vi "Test Host.vi"() -> ()   [LabVIEW 2014]
uses:
  <vilib>/FPGAPlugInAG/PXIe-7962R/niLvFpga_Open_PXIe-7962R.vi
  <vilib>/rvi/interface/common/dynamic/niFpgaDynamicAddResources.vi
  <vilib>/LabVIEW Targets/FPGA/FlexRIO/CustomFPGAMethods/79XXR_Method_IOModuleStatusImpl.vi
  <vilib>/Utility/error.llb/Error Cluster From Error Code.vi
  <vilib>/rvi/errors/niLvFpgaAdjustHostInterfaceError.vi
  <vilib>/rvi/interface/common/niFpgaWaitOnOcc.vi
  <instrlib>/_niInstr/Streaming/v1/Host/Public/Start Finite Stream.vi
  <instrlib>/_niInstr/Streaming/v1/Host/Public/Wait for Stream.vi
  <vilib>/FPGAPlugInAG/Dynamic/niLvFpga_Close_Dynamic.vi
  <vilib>/rvi/interface/nirviOpenFPGA/nirviOpenFPGA.xnode
  FPGA Bitfiles/MochiFPGAControl_FPGATarget_pxie7962fpga_vH47uBXjtQs.lvbitx
  pxie_7962_fpga.vi
  <vilib>/rvi/interface/nirviMethod/nirviMethod.xnode
  <vilib>/rvi/interface/nirviReadWriteControl/nirviReadWriteControl.xnode
  <vilib>/rvi/interface/nirviCloseFPGA/nirviCloseFPGA.xnode
  <instrlib>/_niInstr/Streaming/v1/Host/niInstr Streaming v1 Host.lvlib
  <vilib>/rvi/errors/niLvFpgaMergeErrorWithErrorCode.vi
  <vilib>/rvi/interface/Simulation/niFpgaSimulationCallBeginRW.vi
  NiFpgaLv.dll
  <vilib>/FPGAPlugInAG/Dynamic/niLvFpga_ReadFifo_Dynamic.vi
  <vilib>/FPGAPlugInAG/Dynamic/niLvFpga_ConfigureFifo_Dynamic.vi
  <vilib>/FPGAPlugInAG/Dynamic/niLvFpga_StartFifo_Dynamic.vi
panel:
  out "Bits out DRAM":u64
  out "Writes to DRAM":u64
  in  "?":enum32{"AI 0", "All AI"}(tab)
  out "AI 0":dbl[](graph)
  out "All AI":dbl[][](graph)
  in  "Debug":bool
  out "Bits out DMA":u64
  out "Bits aquired":u64
  out "Writes to DMA":u64
  out "Samples Aquired":u64
  out "Voltage":dbl[][](array[numeric])
  out "Counts":i16[][](array[numeric])
  out "error out":errorcluster
  out "samples transferred":u64
  in  "stop":bool
  out "Raw DMA readout":u64[](array[numeric])
  in  "num samples":u64=64000
  in  "Go":bool
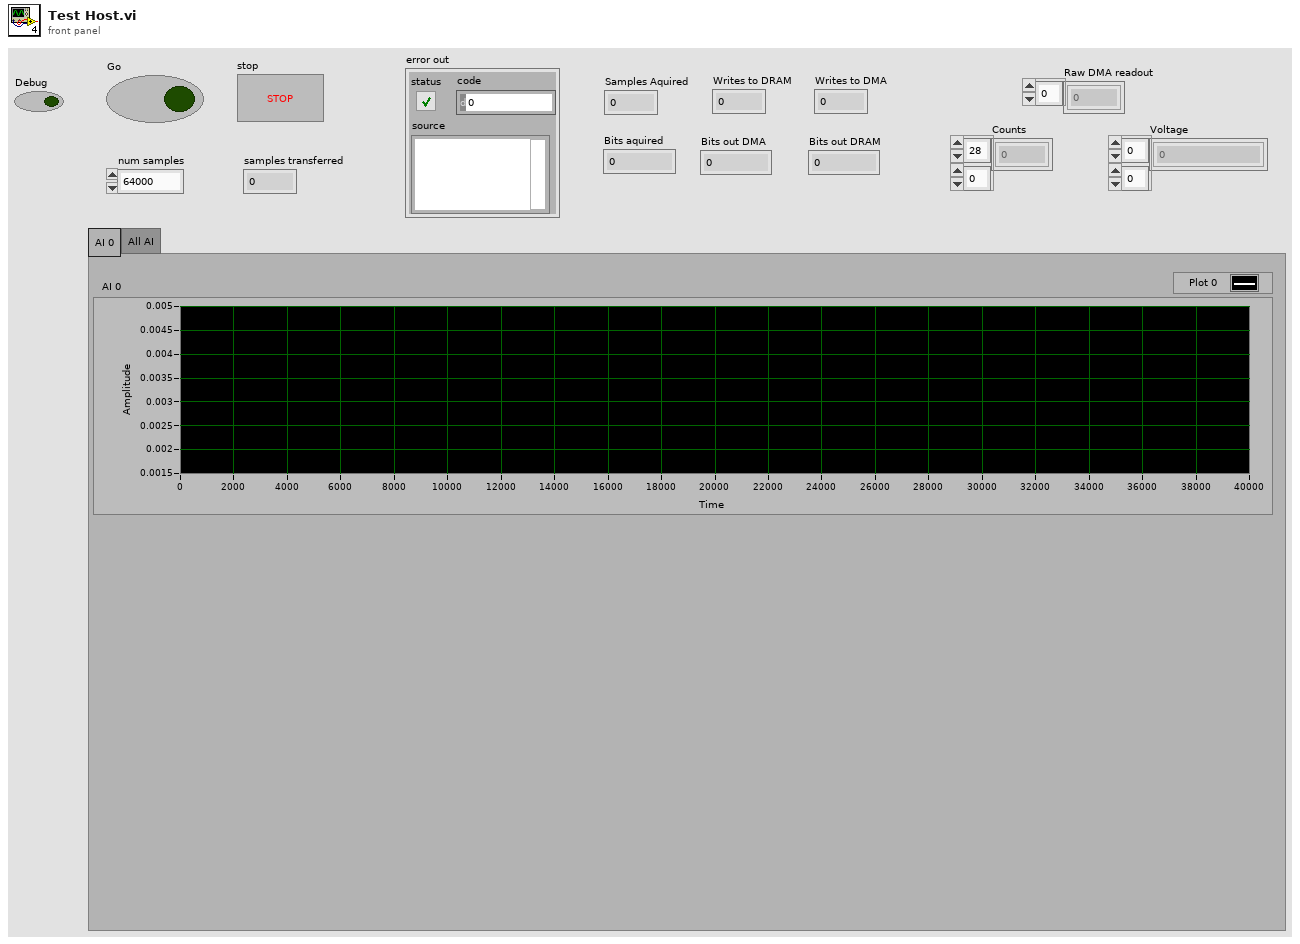
[diagram p1: front panel]
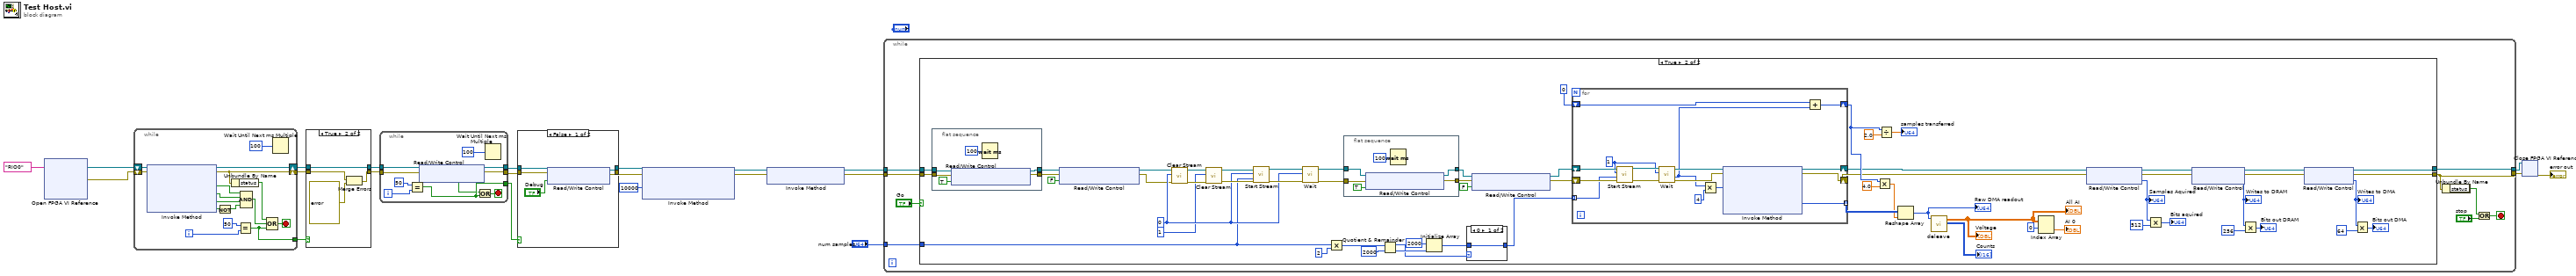
[diagram p0: block diagram]
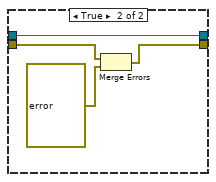
[diagram p2: hidden frame]
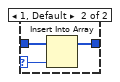
[diagram p5: hidden frame]
diagram:
  n1 = xnode "Open FPGA VI Reference"("resource name"=tag "RIO0") -> ("FPGA VI Reference Out"=w4:refnum<k20>, "error out"=w5:errorcluster)  [unwired: 1 in]
  n2 = while {
    shift-right: [w29] -> w12
    shift-left: w5 -> [w37]
    shift-right: [w36] -> w10
    shift-left: w4 -> [w38]
    tunnel: [w25] -> w11
    i -> [w31]
    stop <- w26 stop-if-true
    n3 = xnode "Invoke Method"("FPGA VI Reference In"=w38, "error in"=w37) -> ("FPGA VI Reference Out"=w36:refnum<k20>, "error out"=w29:errorcluster, "IO Module Present?"=w35:bool, "Power Enabled?"=w34:bool, "IO Enabled?"=w33:bool, "IO Module Mismatch?"=w24:bool)
    n4 = Not(x=w24) -> (.not. x?=w23:bool)
    n5 = Unbundle By Name(w29) -> ("status"=w28:bool)
    n6 = Equal?(x=50, y=w31) -> (x = y?=w25:bool)
    n7 = Compound Arithmetic op=AND(w35, w34, w33, w23) -> (w27:bool)
    n8 = Compound Arithmetic op=OR(w28, w27, w25) -> (w26:bool)
    n9 = Wait Until Next ms Multiple(millisecond multiple=u32 100) -> ()  [unwired: 1 out]
  }
  n10 = case shown="True" w11 {
    tunnel: w12 -> [w39 w43]
    tunnel: [w39 w42] -> w8
    tunnel: w10 -> [w40 w41]
    tunnel: [w40 w41] -> w9
    frame False {
    }
    frame True {
      n11 = Merge Errors(w43, errorcluster {"status"=TRUE, "code"=-1, "source"="The IO Module was not present, powered, or the IO were not enabled.  Verify the NI 5752 is securly connected and try again."} ("error in")) -> (w42:errorcluster)
    }
  }
  n12 = while {
    tunnel: w9 -> [w49]
    tunnel: [w46] -> w2
    tunnel: [w47] -> w1
    tunnel: [w50] -> w3
    tunnel: w8 -> [w48]
    i -> [w53]
    stop <- w51 stop-if-true
    n13 = Equal?(x=50, y=w53) -> (x = y?=w50:bool)
    n14 = xnode "Read/Write Control"("FPGA VI Reference In"=w49, "error in"=w48) -> ("FPGA VI Reference Out"=w46:refnum<k20>, "error out"=w47:errorcluster, "IO Module Init Done"=w45:bool)
    n15 = Or(x=w45, y=w50) -> (x .or. y?=w51:bool)
    n16 = Wait Until Next ms Multiple(millisecond multiple=u32 100) -> ()  [unwired: 1 out]
  }
  n17 = case shown="False" w3 {
    tunnel: w1 -> [w56 w62]
    tunnel: [w55 w61] -> w6
    tunnel: w2 -> [w59 w60]
    tunnel: [w58 w60] -> w7
    frame False {
      n18 = xnode "Read/Write Control"("FPGA VI Reference In"=w59, "error in"=w56, "Output Debug Data"="Debug") -> ("FPGA VI Reference Out"=w58:refnum<k20>, "error out"=w55:errorcluster)
    }
    frame True {
      n19 = Merge Errors(w62, errorcluster {"status"=TRUE, "code"=-1, "source"="The IO Module CLIP was not ready. If you are using any external clocks, make sure they are connected and within the supported specifications."} ("error in")) -> (w61:errorcluster)
    }
  }
  n20 = xnode "Invoke Method"("FPGA VI Reference In"=w7, "error in"=w6, "Requested Depth"=u32 10000) -> ("FPGA VI Reference Out"=w21:refnum<k20>, "error out"=w20:errorcluster)  [unwired: 1 out]
  n21 = xnode "Invoke Method"("FPGA VI Reference In"=w21, "error in"=w20) -> ("FPGA VI Reference Out"=w19:refnum<k20>, "error out"=w18:errorcluster)
  n22 = while {
    tunnel: w19 -> [w71]
    tunnel: w18 -> [w67]
    tunnel: "num samples" -> [w70]
    tunnel: [w69] -> w14
    tunnel: [w66] -> w16
    stop <- w68 stop-if-true
    n23 = case shown="True" "Go" {
      tunnel: w71 -> [w74 w109]
      tunnel: w70 -> [_ w86]
      tunnel: [w74 w77] -> w69
      tunnel: w67 -> [w73 w76]
      tunnel: [w73 w75] -> w66
      frame False {
        (unwired) errorcluster {"status"=FALSE, "code"=0, "source"=""} ("error out")
      }
      frame True {
        w127 = 0 ("stream index")
        n24 = flat-sequence {
          tunnel: [w164] -> w113
          tunnel: w109 -> [w163]
          tunnel: [w162] -> w108
          tunnel: w76 -> [w161]
          frame #0 {
            n25 = xnode "Read/Write Control"("FPGA VI Reference In"=w163, "error in"=w161, "Reset DRAM write address"=TRUE) -> ("FPGA VI Reference Out"=w162:refnum<k20>, "error out"=w164:errorcluster)
            n26 = Wait (ms)(milliseconds to wait=u32 100) -> ()  [unwired: 1 out]
          }
        }
        n27 = xnode "Read/Write Control"("FPGA VI Reference In"=w108, "error in"=w113, "Reset DRAM write address"=FALSE) -> ("FPGA VI Reference Out"=w87:refnum<k20>, "error out"=w93:errorcluster)
        n28 = call <instrlib>:"Clear Stream.vi"("error in (no error)"=w93, "stream index"=w127, "refnum in"=w87) -> ("error out"=w133:errorcluster, "refnum out"=w134:refnum<k20>)  [unwired: 7 in]
        n29 = call <instrlib>:"Clear Stream.vi"("error in (no error)"=w133, "stream index"=1, "refnum in"=w134) -> ("error out"=w131:errorcluster, "refnum out"=w132:refnum<k20>)  [unwired: 7 in]
        n30 = call-poly <instrlib>:"Start Stream.vi"("error in (no error)"=w131, "num samples"=w86, "stream index"=w127, "refnum in"=w132) -> ("error out"=w128:errorcluster, "refnum out"=w129:refnum<k20>)  [unwired: 6 in]
        n31 = call-poly <instrlib>:"Wait.vi"("error in (no error)"=w128, "stream index"=w127, "refnum in"=w129) -> ("error out"=w110:errorcluster, "refnum out"=w107:refnum<k20>)  [unwired: 5 in, 2 out]
        n32 = Multiply(x=w86, y=u64 2) -> (x*y=w99:u64)
        n33 = flat-sequence {
          tunnel: w110 -> [w159]
          tunnel: [w157] -> w111
          tunnel: w107 -> [w156]
          tunnel: [w155] -> w106
          frame #0 {
            n34 = xnode "Read/Write Control"("FPGA VI Reference In"=w156, "error in"=w159, "Reset DRAM read address"=TRUE ("Reset DRAM write address")) -> ("FPGA VI Reference Out"=w155:refnum<k20>, "error out"=w157:errorcluster)
            n35 = Wait (ms)(milliseconds to wait=u32 100) -> ()  [unwired: 1 out]
          }
        }
        n36 = Quotient & Remainder(x=w99, y=u64 2000) -> (x-y*floor(x/y)=w88:u64, floor(x/y)=w97:u64)
        n37 = Initialize Array(u64 2000 ("element"), w97) -> (w95:u64[])
        n38 = case shown="0" w88 {
          selector: w88 -> [_ w136]
          tunnel: w95 -> [w135 w138]
          tunnel: [w135 w137] -> w94
          frame 0 {
          }
          frame 1, Default {
            n39 = Insert Into Array(array=w138, new element=w136) -> (w137:u64[])  [unwired: 1 in]
          }
        }
        n40 = xnode "Read/Write Control"("FPGA VI Reference In"=w106, "error in"=w111, "Reset DRAM read address"=FALSE ("Reset DRAM write address")) -> ("FPGA VI Reference Out"=w100:refnum<k20>, "error out"=w101:errorcluster)
        n41 = for {
          shift-right: [w140] -> w92
          shift-left: w100 -> [w151]
          shift-right: [w139] -> w85
          shift-left: w101 -> [w150]
          shift-right: [w154] -> w103
          shift-left: u64 0 -> [w147]
          tunnel: w94 -> [w148] mode=indexing
          tunnel: [w141] -> w91 mode=indexing
          w149 = 1 ("stream index")
          n42 = call-poly <instrlib>:"Start Stream.vi"("error in (no error)"=w150, "num samples"=w148, "stream index"=w149, "refnum in"=w151) -> ("error out"=w152:errorcluster, "refnum out"=w153:refnum<k20>)  [unwired: 6 in]
          n43 = call-poly <instrlib>:"Wait.vi"("error in (no error)"=w152, "stream index"=w149, "refnum in"=w153) -> ("error out"=w145:errorcluster, "samples transferred"=w143:u64, "refnum out"=w146:refnum<k20>)  [unwired: 5 in, 1 out]
          n44 = Multiply(x=w143, y=u64 4) -> (x*y=w144:u64)
          n45 = xnode "Invoke Method"("FPGA VI Reference In"=w146, "error in"=w145, "Number of Elements"=w144) -> ("FPGA VI Reference Out"=w140:refnum<k20>, "error out"=w139:errorcluster, "Data"=w141:u64[])  [unwired: 1 in, 1 out]
          n46 = Add(x=w147, y=w143) -> (x+y=w154:u64)
        }
        n47 = Multiply(x=w103, y=4.0) -> (x*y=w90:dbl)
        n48 = Divide(x=w103, y=2.0) -> (x/y=→"samples transferred":dbl)
        n49 = Reshape Array(w91, w90) -> (w89:u64[])
        "Raw DMA readout" <- w89
        n50 = call "deleave.vi"("Data"=w89) -> ("Counts"=→"Counts":i16[][], "Voltage"=w116:dbl[][])  [unwired: 9 in]
        "Voltage" <- w116
        "All AI" <- w116
        n51 = Index Array(array=w116, index (row)=0) -> (element=→"AI 0":dbl[])  [unwired: 1 in]
        n52 = xnode "Read/Write Control"("FPGA VI Reference In"=w92, "error in"=w85) -> ("FPGA VI Reference Out"=w81:refnum<k20>, "error out"=w80:errorcluster, "Samples Aquired"=w123:u64)
        "Samples Aquired" <- w123
        n53 = Multiply(x=w123, y=u64 512) -> (x*y=→"Bits aquired":u64)
        n54 = xnode "Read/Write Control"("FPGA VI Reference In"=w81, "error in"=w80) -> ("FPGA VI Reference Out"=w79:refnum<k20>, "error out"=w78:errorcluster, "Writes to DRAM"=w83:u64)
        "Writes to DRAM" <- w83
        n55 = Multiply(x=w83, y=u64 256) -> (x*y=→"Bits out DRAM":u64)
        n56 = xnode "Read/Write Control"("FPGA VI Reference In"=w79, "error in"=w78) -> ("FPGA VI Reference Out"=w77:refnum<k20>, "error out"=w75:errorcluster, "Writes to DMA"=w120:u64)
        "Writes to DMA" <- w120
        n57 = Multiply(x=w120, y=u64 64) -> (x*y=→"Bits out DMA":u64)
      }
    }
    n58 = Unbundle By Name(w66) -> ("status"=w64:bool)
    n59 = Or(x=w64, y="stop") -> (x .or. y?=w68:bool)
  }
  n60 = xnode "Close FPGA VI Reference"("FPGA VI Reference In"=w14, "error in"=w16) -> ("error out"=→"error out":errorcluster)
